vi "Pre Launch Init.vi"(11 "Base UI Actor in":refnum<class "Base UI Actor.lvclass">) -> (0 "error out":errorcluster, 3 "Base UI Actor out":refnum<class "Base UI Actor.lvclass">)   [LabVIEW 2017, in "Assert API Components.lvlib" / "Base UI Actor.lvlib" / "Base UI Actor.lvclass"]
doc: "(<B>Filename</B>: Actor Framework.lvlib:Actor.lvclass:Pre Launch Init.vi)\n\nDefines behavior that occurs after the Launch Nested Actor method is invoked but before the actor's Actor Core method begins running.\n\nBy default, this method does nothing. A descendant class may override it to define behavior."
uses:
  Base UI Actor.lvclass
  Base UI Actor.lvclass/Base UI Actor.ctl
  <vilib>/ActorFramework/Actor/Actor.lvclass
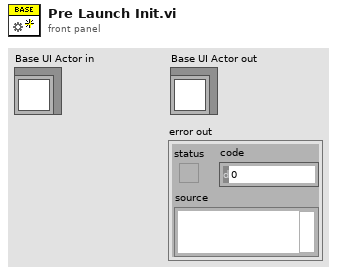
[diagram p1: front panel]
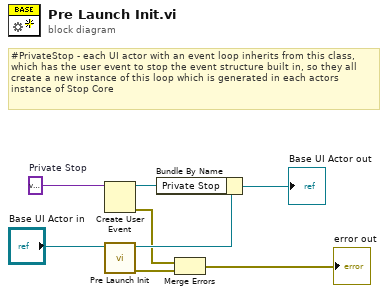
[diagram p0: block diagram]
diagram:
  w5 = variant  # Private Stop
  # "#PrivateStop - each UI actor with an event loop inherits from this class, which has the user event to stop the event structure built in, so they all create a new instance of this loop which is generated in each actors instance of Stop Core"
  n1 = Create User Event(user event datatype=w5) -> (user event=w3:refnum<user-event>, error out=w1:errorcluster)  [unwired: 1 in]
  n2 = call-parent "Pre Launch Init.vi"("Actor in"="Base UI Actor in") -> ("error out"=w8:errorcluster, "Actor out"=w7:refnum<class "Base UI Actor.lvclass">)  [unwired: 9 in]
  n3 = Bundle By Name(cluster=w7, "Private Stop"=w3) -> (→"Base UI Actor out":refnum<class "Base UI Actor.lvclass">)
  n4 = Merge Errors(w1, w8) -> (→"error out":errorcluster)
